vi "Row Check.vi"(8 "error in (no error)":errorcluster caption="错误输入（无错误）", 11 "listbox 输入":refnum<class "listbox.lvclass">) -> (0 "error out":errorcluster caption="错误输出", 2 "为空？":bool, 3 "listbox 输出":refnum<class "listbox.lvclass">)   [LabVIEW 2016, in "listbox.lvclass"]
uses:
  listbox.lvclass
  listbox.lvclass/listbox.ctl
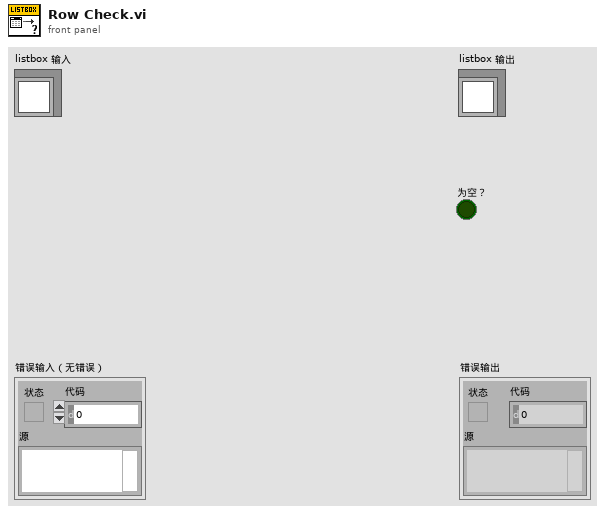
[diagram p1: front panel]
types:
  T1 = typedef "LVRowAndColumnTypeDef.ctl" = cluster{"Row":i32, "Column":i32}
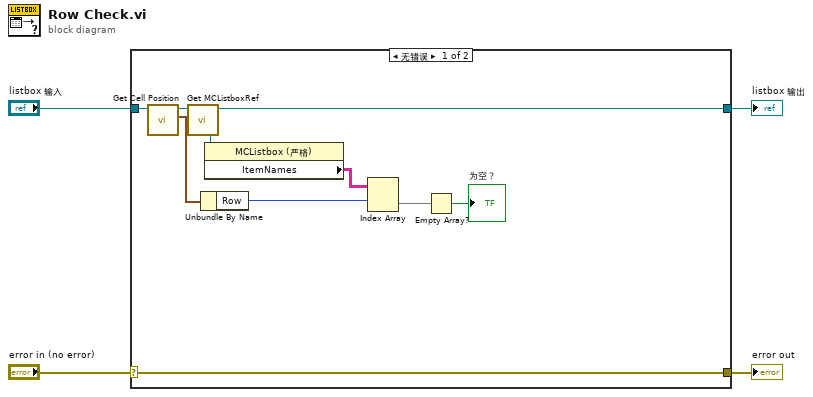
[diagram p0: block diagram]
diagram:
  n1 = case shown="无错误" "error in (no error)" {
    selector: "error in (no error)" -> [w13 w16]
    tunnel: [w13 w16] -> w3
    tunnel: [w10 w15] -> w1
    tunnel: "listbox 输入" -> [w14 w15]
    frame No Error {
      n2 = call "Get Cell Position.vi"("listbox in"=w14) -> ("Cell Position"=w6:T1, "listbox out"=w11:refnum<class "listbox.lvclass">)  [unwired: 9 in]
      n3 = call "Get MCListboxRef.vi"("listbox in"=w11) -> ("MCListboxRef"=w9:refnum<vi>, "listbox out"=w10:refnum<class "listbox.lvclass">)  [unwired: 9 in]
      n4 = Unbundle By Name(w6) -> ("Row"=w5:i32)
      n5 = property class="MCListbox (严格)"(reference=w9) -> ("ItemNames"=w8:string[][])  [unwired: 1 in, 2 out]
      n6 = Index Array(array=w8, index (row)=w5) -> (element=w7:string[])  [unwired: 1 in]
      n7 = Empty Array?(array=w7) -> (empty?=→"为空？":bool)
    }
    frame Error {
    }
  }
  "error out" <- w3
  "listbox 输出" <- w1
